vi "FTW-XML-Construct.vi"(5 "XML String":string, 11 "error in":errorcluster) -> (4 "XML Document":refnum<k20>, 15 "error out":errorcluster)   [LabVIEW 2014]
uses:
  core/error/FTW-ERR-NoErrorConstant.vi
  core/error/FTW-ERR-CallChain.vi
  core/string/FTW-STR-ReplaceWhitespace.vi
  <resource>/objmgr/DOMUserDefRef.rc
  DOMUserDefRef.dll
panel:
  # "Inputs"
  # "Outputs"
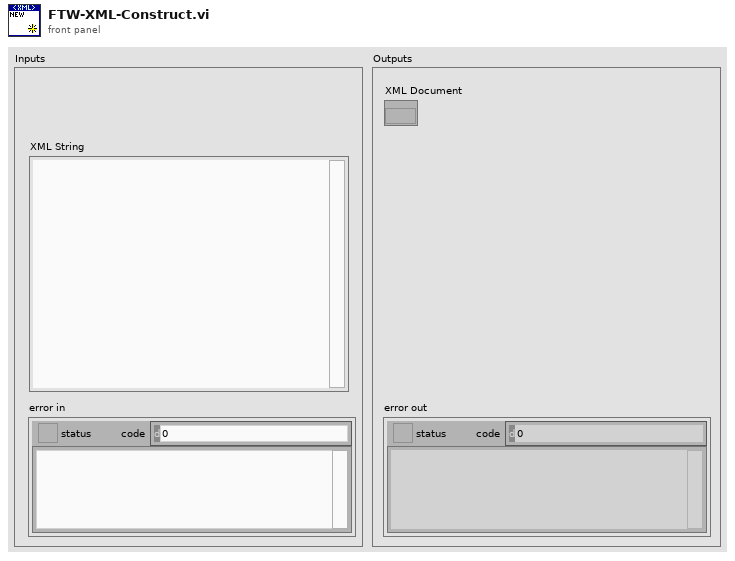
[diagram p1: front panel]
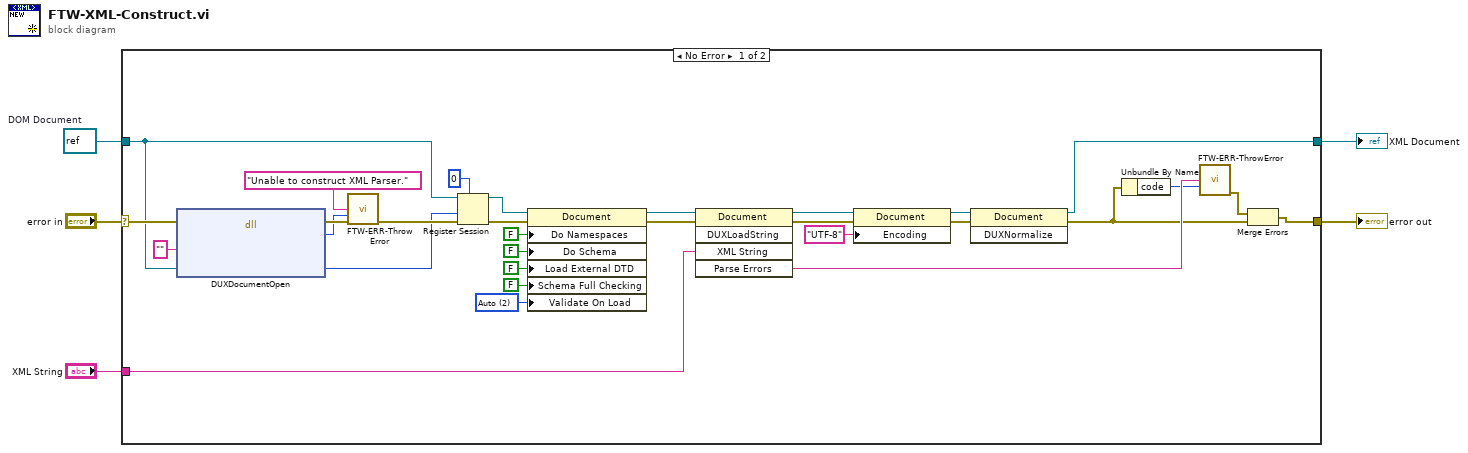
[diagram p0: block diagram]
diagram:
  w1 = refnum<k20> refnum  # DOM Document
  n1 = case shown="No Error" "error in" {
    selector: "error in" -> [w35 w37]
    tunnel: [w21 w37] -> w5
    tunnel: [w12 w36] -> w3
    tunnel: "XML String" -> [w25 _]
    tunnel: w1 -> [w20 w36]
    frame No Error {
      w28 = 2 items=["Never", "Always", "Auto"] ("Validate On Load")
      n2 = dll-call lib="DOMUserDefRef.*" fn="DUXDocumentOpen"(error in=w35, "Name"="", "Document Session"=w20) -> (error out=w19:errorcluster, "Return"=w16:i32, "Document Session"=w15:u64)  [unwired: 2 in, 2 out]
      n3 = call "FTW-ERR-ThrowError.vi"("Error Message"="Unable to construct XML Parser.", "Error Code"=w16, "error in"=w19) -> ("error out"=w18:errorcluster)  [unwired: 12 in]
      n4 = Register Session(7:0 ("cleanup mode (default to class = 0)"), 8:w18, 9:w15, 11:w20) -> (0:w33:errorcluster, 3:w34:refnum<k20>)  [unwired: 1 in]
      n5 = property class="Document"(reference=w34, error in=w33, "Do Namespaces"=FALSE ("Process Namespaces"), "Do Schema"=FALSE ("Process Schema"), "Load External DTD"=FALSE, "Schema Full Checking"=FALSE, "Validate On Load"=w28) -> (reference out=w26:refnum<k20>, error out=w27:errorcluster)
      n6 = invoke class="Document" method="DUXLoadString"(reference=w26, error in=w27, "XML String"=w25) -> (reference out=w10:refnum<k20>, error out=w9:errorcluster, "Parse Errors"=w24:string)  [unwired: 2 in, 2 out]
      n7 = property class="Document"(reference=w10, error in=w9, "Encoding"="UTF-8" ("Document Encoding")) -> (reference out=w8:refnum<k20>, error out=w7:errorcluster)
      n8 = invoke class="Document" method="DUXNormalize"(reference=w8, error in=w7) -> (reference out=w12:refnum<k20>, error out=w11:errorcluster)  [unwired: 1 in, 1 out]
      n9 = Unbundle By Name(w11) -> ("code"=w23:i32)
      n10 = call "FTW-ERR-ThrowError.vi"("Error Message"=w24, "Error Code"=w23) -> ("error out"=w22:errorcluster)  [unwired: 13 in]
      n11 = Merge Errors(w22, w11) -> (w21:errorcluster)
    }
    frame Error {
    }
  }
  "error out" <- w5
  "XML Document" <- w3
